vi "Close.vi"(8 "error in (no error)":errorcluster, 11 "G-UE in":refnum<class "G-UE.lvclass">) -> (0 "error out":errorcluster, 3 "G-UE out":refnum<class "G-UE.lvclass">)   [LabVIEW 2016, in "G-UE.lvclass"]
uses:
  G-UE.lvclass
  G-UE.lvclass/G-UE.ctl
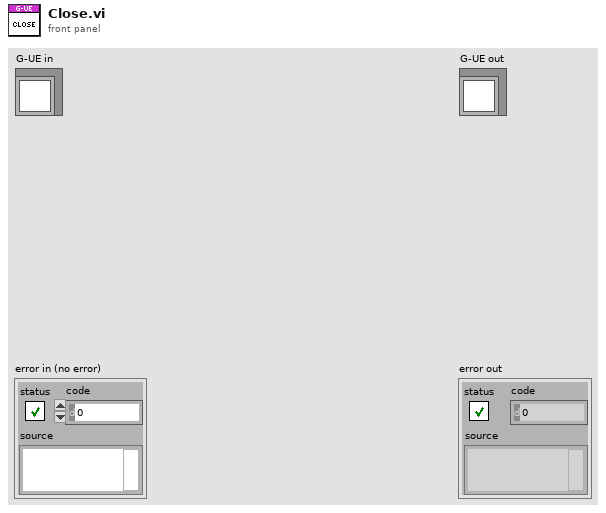
[diagram p1: front panel]
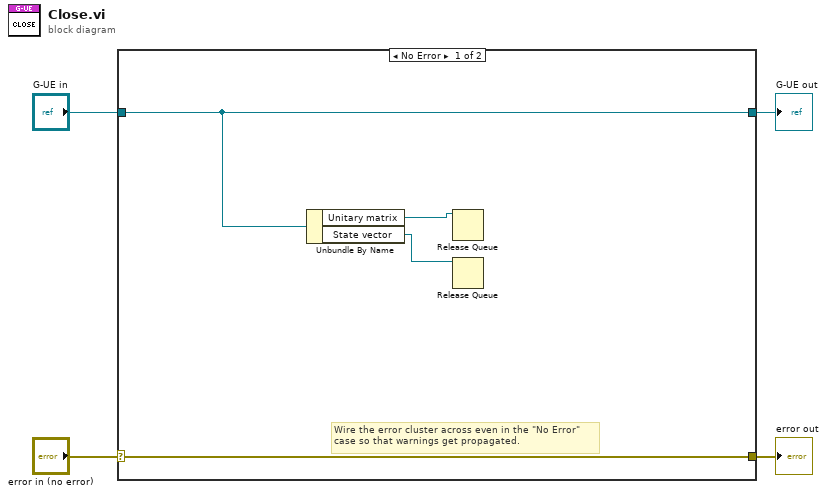
[diagram p0: block diagram]
diagram:
  n1 = case shown="No Error" "error in (no error)" {
    selector: "error in (no error)" -> [w8 w10]
    tunnel: [w8 w10] -> w3
    tunnel: [w5 w9] -> w1
    tunnel: "G-UE in" -> [w5 w9]
    frame No Error {
      # "Wire the error cluster across even in the \"No Error\"\ncase so that warnings get propagated."
      n2 = Unbundle By Name(w5) -> ("Unitary matrix"=w6:refnum<queue>, "State vector"=w7:refnum<queue>)
      n3 = Release Queue(queue=w6) -> ()  [unwired: 2 in, 3 out]
      n4 = Release Queue(queue=w7) -> ()  [unwired: 2 in, 3 out]
    }
    frame Error {
    }
  }
  "error out" <- w3
  "G-UE out" <- w1
